vi "HFRR ADV v03.vi"() -> ()   [LabVIEW 2025] (continued)
            n807 = call "CAMERA LIVE FEED FGV.vi"("Enum - Menu"=CAMERA_LIVE_FEED_ENUM."CAMERA MINIMIZE") -> ()  [unwired: 9 in, 2 out]
          }
        }
        n808 = local write "CAMERA ROI MAX TEMP"(TRUE ("CAMERA ROI MAX TEMP")) -> ()
        n809 = case shown="True" w1172 {
          selector: w1172 -> [_ w1178]
          frame False {
          }
          frame True {
            n810 = Not(x=w1178) -> (.not. x?=w1177:bool)
            n811 = local write "CAMERA ROI MIN TEMP"(w1177) -> ()
            n812 = call "IMAGE ANALYSIS.vi"("Enum"=POST_ANALYSIS_ENUM."MINIMIZE UI") -> ()  [unwired: 9 in, 2 out]
          }
        }
      }
      frame "Mooha" {
        n813 = local read "LIVE FEED MIN TEMP"() -> (w1184:bool)
        n814 = local write "LIVE FEED MAX TEMP"(TRUE ("LIVE FEED MAX TEMP")) -> ()
        n815 = local read "CAMERA ROI MIN TEMP"() -> (w1182:bool)
        n816 = case shown="True" w1184 {
          selector: w1184 -> [_ w1191]
          frame False {
          }
          frame True {
            n817 = Not(x=w1191) -> (.not. x?=w1190:bool)
            n818 = local write "LIVE FEED MIN TEMP"(w1190) -> ()
            n819 = call "CAMERA LIVE FEED FGV.vi"("Enum - Menu"=CAMERA_LIVE_FEED_ENUM."CAMERA MINIMIZE") -> ()  [unwired: 9 in, 2 out]
          }
        }
        n820 = local write "CAMERA ROI MAX TEMP"(TRUE ("CAMERA ROI MAX TEMP")) -> ()
        n821 = case shown="True" w1182 {
          selector: w1182 -> [_ w1188]
          frame False {
          }
          frame True {
            n822 = Not(x=w1188) -> (.not. x?=w1187:bool)
            n823 = local write "CAMERA ROI MIN TEMP"(w1187) -> ()
            n824 = call "IMAGE ANALYSIS.vi"("Enum"=POST_ANALYSIS_ENUM."MINIMIZE UI") -> ()  [unwired: 9 in, 2 out]
          }
        }
      }
    }
    n825 = local read "Auto Start Test"() -> (w933:bool)
    n826 = case shown="True" "sign in temp" {
      frame False {
      }
      frame True {
        w970 = 1 ("y")
        n827 = local read "USERNAME"() -> (w976:string)
        n828 = local read "USER ID"() -> (w973:string)
        n829 = call <vilib>:"Trim Whitespace.vi"("string"=w976) -> ("trimmed string"=w975:string)  [unwired: 1 in]
        n830 = call <vilib>:"Trim Whitespace.vi"("string"=w973) -> ("trimmed string"=w974:string)  [unwired: 1 in]
        n831 = String Length(string=w975) -> (length=w972:i32)
        n832 = String Length(string=w974) -> (length=w971:i32)
        n833 = Greater?(x=w972, y=w970) -> (0:w969:bool)
        n834 = Greater?(x=w971, y=w970) -> (0:w968:bool)
        n835 = And(x=w969, y=w968) -> (x .and. y?=w967:bool)
        n836 = case shown="True" w967 {
          frame False {
            n837 = property on="Sign In" class="Bool (strict)"("DisabledEnum"=T13."Disabled" ("Disabled")) -> ()  [unwired: 2 in, 2 out]
          }
          frame True {
            n838 = property on="Sign In" class="Bool (strict)"("DisabledEnum"=T13."Enabled" ("Disabled")) -> ()  [unwired: 2 in, 2 out]
          }
        }
      }
    }
    n839 = local read "Air Temperature"() -> (w950:bool)
    n840 = local read "Coefficient Of Friction"() -> (w951:bool)
    n841 = case shown="False" w933 {
      frame False {
        n842 = local read "Auto stop temp"() -> (w964:bool)
        n843 = case shown="True" w964 {
          frame False {
          }
          frame True {
            n844 = local write "Auto Start Temp"(FALSE ("Auto Start Temp")) -> ()
          }
        }
      }
      frame True {
        "Auto stop temp" <- TRUE ("Auto stop temp")
      }
    }
    n845 = local read "Humidity"() -> (w949:bool)
    n846 = case shown="\"HOME\"" w961 {
      frame "HOME" {
        n847 = local write "main tab sub"(enum32{"Page 1", "Page 2"}."Page 1" ("main tab sub")) -> ()
      }
      frame Default {
        n848 = local write "main tab sub"(enum32{"Page 1", "Page 2"}."Page 2" ("main tab sub")) -> ()
      }
    }
    n849 = case shown="True" w960 {
      selector: w960 -> [_ w1296]
      frame False {
      }
      frame True {
        n850 = Not(x=w1296) -> (.not. x?=w1295:bool)
        n851 = local write "Sign In"(w1295) -> ()
        n852 = local write "Main Dashboard Buttons"(T1."Test Setup" ("Main Dashboard Buttons")) -> ()
      }
    }
    n853 = case shown="\"Numeric Display\", Default" "Num/Graph" {
      frame "Numeric Display", Default {
        n854 = property on="Single/Multiple" class="RadioBtnsControl (strict)"("Visible"=FALSE) -> ()  [unwired: 2 in, 2 out]
        n855 = property on="Single - Graph" class="Ring (strict)"("Visible"=FALSE) -> ()  [unwired: 2 in, 2 out]
        n856 = local write "Main Tab Display"(T4."Dashboard 1" ("Main Tab Display")) -> ()
      }
      frame "Graph Display" {
        n857 = property on="Single/Multiple" class="RadioBtnsControl (strict)"("Visible"=TRUE) -> ()  [unwired: 2 in, 2 out]
        n858 = case shown="\"Multiple\"" "Single/Multiple" {
          frame "Single ", Default {
            n859 = property on="Single - Graph" class="Ring (strict)"("Visible"=TRUE) -> ()  [unwired: 2 in, 2 out]
            n860 = local write "Main Tab Display"(T4."Dashboard 3" ("Main Tab Display")) -> ()
          }
          frame "Multiple" {
            n861 = property on="Single - Graph" class="Ring (strict)"("Visible"=FALSE) -> ()  [unwired: 2 in, 2 out]
            n862 = local write "Main Tab Display"(T4."Dashboard 2" ("Main Tab Display")) -> ()
          }
        }
      }
    }
    n863 = local read "Stroke"() -> (w948:bool)
    n864 = local read "USERNAME"() -> (w954:string)
    n865 = local read "USER ID"() -> (w953:string)
    n866 = case shown="True" w951 {
      selector: w951 -> [_ w1231]
      frame False {
      }
      frame True {
        n867 = Not(x=w1231) -> (.not. x?=w1230:bool)
        n868 = local write "Coefficient Of Friction"(w1230) -> ()
        n869 = local write "Tab Control 2"(T6."Coefficient Of Friction" ("Tab Control 2")) -> ()
      }
    }
    n870 = case shown="True" w950 {
      selector: w950 -> [_ w1228]
      frame False {
      }
      frame True {
        n871 = Not(x=w1228) -> (.not. x?=w1226:bool)
        n872 = local write "Air Temperature"(w1226) -> ()
        n873 = local write "Tab Control 2"(T6."Air Temperature" ("Tab Control 2")) -> ()
      }
    }
    n874 = local write "Operator ID"(w953) -> ()
    n875 = case shown="True" w948 {
      selector: w948 -> [_ w1222]
      frame False {
      }
      frame True {
        n876 = Not(x=w1222) -> (.not. x?=w1220:bool)
        n877 = local write "Stroke"(w1220) -> ()
        n878 = local write "Tab Control 2"(T6."Stroke" ("Tab Control 2")) -> ()
      }
    }
    n879 = local write "tested by"(w954) -> ()
    n880 = case shown="True" w949 {
      selector: w949 -> [_ w1225]
      frame False {
      }
      frame True {
        n881 = Not(x=w1225) -> (.not. x?=w1223:bool)
        n882 = local write "Humidity"(w1223) -> ()
        n883 = local write "Tab Control 2"(T6."Humidity" ("Tab Control 2")) -> ()
      }
    }
    n884 = case shown="\"Advance\"" "Main Dashboard Buttons" {
      tunnel: [T2."HOME" ("Main Tab") T2."Test Setup" ("Main Tab") T2."Acquire" ("Main Tab") T2."Adv Scar" ("Main Tab") T2."Adv Scar Report" ("Main Tab") T2."Compare Files" ("Main Tab") T2."About" ("Main Tab") T2."Advance" ("Main Tab")] -> w958
      frame "Home", Default {
      }
      frame "Test Setup" {
      }
      frame "Dashboard" {
      }
      frame "Imaging" {
      }
      frame "Report" {
      }
      frame "Analysis" {
      }
      frame "About" {
      }
      frame "Advance" {
      }
    }
    n885 = Wait (ms)(milliseconds to wait=u32 100) -> ()  [unwired: 1 out]
    n886 = local read "Main Tab Display"() -> (w952:T4)
    n887 = local write "Main Tab"(w958) -> ()
    n888 = case shown="\"Dashboard 3\"" w952 {
      frame "Dashboard 1", Default {
        n889 = property on="Reset Graph" class="Bool (strict)"("Visible"=FALSE) -> ()  [unwired: 2 in, 2 out]
      }
      frame "Dashboard 2" {
        n890 = property on="Reset Graph" class="Bool (strict)"("Visible"=TRUE) -> ()  [unwired: 2 in, 2 out]
      }
      frame "Dashboard 3" {
        n891 = property on="Reset Graph" class="Bool (strict)"("Visible"=TRUE) -> ()  [unwired: 2 in, 2 out]
      }
    }
    n892 = local read "SCAR MEASURMENT"() -> (w940:enum32{"Auto Scar", "Manual Scar"})
    n893 = local read "Humidity"() -> (w955:bool)
    n894 = local read "Cap Live Image"() -> (w937:bool)
    n895 = local read "Sample Temperature"() -> (w947:bool)
    n896 = local read "Air Temp vs Humidity"() -> (w945:bool)
    n897 = local read "Frequency"() -> (w946:bool)
    n898 = case shown="False" w955 {
      frame False {
        n899 = local write "Humidity On Command"(TRUE ("Humidity On Command")) -> ()
        n900 = case shown="True" "Humidity Off Command" {
          selector: "Humidity Off Command" -> [_ w1238]
          frame False {
          }
          frame True {
            n901 = stacked-sequence {
              frame #0 {
                n902 = local read "WriteHumidity"() -> (w1240:string[])
                n903 = Insert Into Array(array=w1240, new element="R;1" ("new element/subarray")) -> (w1241:string[])  [unwired: 1 in]
                n904 = local write "WriteHumidity"(w1241) -> ()
              }
              frame #1 {
                n905 = Wait (ms)(milliseconds to wait=u32 2000) -> ()  [unwired: 1 out]
              }
              frame #2 {
                n906 = local read "EVENT LOG"() -> (w1247:string)
                n907 = local read "WriteHumidity"() -> (w1244:string[])
                n908 = call "Event Log.vi"("Content"="Humidity Control Off" ("string"), "EVENT LOG"=w1247) -> ("EVENT LOG"=w1248:string)  [unwired: 8 in, 1 out]
                n909 = local write "EVENT LOG"(w1248) -> ()
                n910 = Insert Into Array(array=w1244, new element="R;1" ("new element/subarray")) -> (w1245:string[])  [unwired: 1 in]
                n911 = local write "WriteHumidity"(w1245) -> ()
              }
            }
            n912 = Not(x=w1238) -> (.not. x?=w1237:bool)
            n913 = local write "Humidity Off Command"(w1237) -> ()
          }
        }
      }
      frame True {
        n914 = local write "Humidity Off Command"(TRUE ("Humidity Off Command")) -> ()
        n915 = case shown="False" "Humidity On Command" {
          selector: "Humidity On Command" -> [_ w1252]
          frame False {
          }
          frame True {
            n916 = stacked-sequence {
              frame #0 {
                n917 = local read "Set Rh"() -> (w1258:dbl)
                n918 = Number To Fractional String(number=w1258, precision (6)=i16 2) -> (F-format string=w1259:string)  [unwired: 2 in]
                n919 = local read "WriteHumidity"() -> (w1256:string[])
                n920 = Concatenate Strings("M;" ("new element/subarray"), w1259) -> (w1257:string)
                n921 = Insert Into Array(array=w1256, new element=w1257) -> (w1255:string[])  [unwired: 1 in]
                n922 = local write "WriteHumidity"(w1255) -> ()
              }
              frame #1 {
                n923 = Wait (ms)(milliseconds to wait=u32 1500) -> ()  [unwired: 1 out]
              }
              frame #2 {
                (unwired) "% RH" ("string")
                (unwired) i16 2 ("precision (6)")
                (unwired) "M;" ("new element/subarray")
                n924 = local read "Set Rh"() -> (w1266:dbl)
                n925 = Number To Fractional String(number=w1266, precision (6)=i16 2) -> (F-format string=w1263:string)  [unwired: 2 in]
                n926 = local read "WriteHumidity"() -> (w1268:string[])
                n927 = Concatenate Strings("M;" ("new element/subarray"), w1263) -> (w1267:string)
                n928 = Concatenate Strings("Humidity Set to : " ("string"), w1263, "% RH" ("string")) -> (w1261:string)
                n929 = Insert Into Array(array=w1268, new element=w1267) -> (w1269:string[])  [unwired: 1 in]
                n930 = disable-structure shown="Enabled" {
                  frame Enabled {
                    n931 = local read "EVENT LOG"() -> (w1272:string)
                    n932 = call "Event Log.vi"("Content"="Humidity Control On", "EVENT LOG"=w1272) -> ("EVENT LOG"=w1273:string)  [unwired: 8 in, 1 out]
                    n933 = local write "EVENT LOG"(w1273) -> ()
                  }
                  frame Disabled {
                  }
                }
                n934 = disable-structure shown="Enabled" {
                  disable-tunnel: w1261 -> [_ _]
                  frame Enabled {
                    n935 = local read "EVENT LOG"() -> (w1275:string)
                    n936 = call "Event Log.vi"("Content"="Humidity Control On", "EVENT LOG"=w1275) -> ("EVENT LOG"=w1276:string)  [unwired: 8 in, 1 out]
                    n937 = local write "EVENT LOG"(w1276) -> ()
                  }
                  frame Disabled {
                  }
                }
                n938 = local write "WriteHumidity"(w1269) -> ()
              }
            }
            n939 = Not(x=w1252) -> (.not. x?=w1251:bool)
            n940 = local write "Humidity On Command"(w1251) -> ()
          }
        }
      }
    }
    n941 = Equal?(x=w940, y=enum32{"Auto Scar", "Manual Scar"}."Auto Scar" ("SCAR MEASURMENT")) -> (x = y?=w936:bool)
    n942 = local read "TEST STANDARD"() -> (w943:T3)
    n943 = And(x=w937, y=w936) -> (x .and. y?=w938:bool)
    n944 = case shown="True" w938 {
      selector: w938 -> [_ w1037]
      tunnel: errorcluster {"status"=FALSE, "code"=0, "source"=""} ("error in (no error) 3") -> [_ w1038]
      frame False {
      }
      frame True {
        n945 = stacked-sequence {
          tunnel: w1038 -> [_ _ _ _ _ _ _ w1086]
          tunnel: w1037 -> [_ _ _ _ _ w1067 _ _]
          frame #0 {
            n946 = call "CAMERA LIVE FEED FGV.vi"("Enum - Menu"=CAMERA_LIVE_FEED_ENUM."CAMERA MINIMIZE") -> ()  [unwired: 9 in, 2 out]
          }
          frame #1 {
            n947 = property on="Auto Scar Check  2" class="Clust (strict)"("Visible"=TRUE) -> ()  [unwired: 2 in, 2 out]
          }
          frame #2 {
            n948 = String To Path(string="C:\\LAB-IQ\\Image Calibrate v01.dcf") -> (path=w1043:path)
            n949 = Open/Create/Replace File ("Open File")(file path (use dialog)=w1043) -> (refnum out=w1044:refnum<file>)  [unwired: 5 in, 2 out]
            n950 = for {
              N: 4 -> [_]
              tunnel: w1044 -> [w1050]
              i -> [w1046]
              n951 = Read from Text File ("Read File")(file (use dialog)=w1050) -> (text=w1051:string)  [unwired: 3 in, 3 out]
              n952 = String Subset(string=w1051, offset (0)=6, length (rest)=10 ("length (rest)")) -> (substring=w1047:string)
              n953 = Fract/Exp String To Number(string=w1047) -> (number=w1045:dbl)  [unwired: 3 in, 1 out]
              n954 = case shown="0" w1046 {
                tunnel: w1045 -> [w1052 w1053 _ w1054 _]
                frame 0 {
                  "5x Gain" <- w1052
                }
                frame 1 {
                  "10x Gain" <- w1053
                }
                frame 2 {
                }
                frame 3 {
                  "100x gain" <- w1054
                }
                frame 4, Default {
                }
              }
            }
          }
          frame #3 {
            n955 = local read "FILE 3"() -> (w1060:string)
            n956 = call <vilib>:"Trim Whitespace.vi"("string"="C:\\LAB-IQ\\images\\") -> ("trimmed string"=w1062:string)  [unwired: 1 in]
            n957 = String To Path(string=w1062) -> (path=w1061:path)
            n958 = Concatenate Strings(w1060, ".png" ("string")) -> (w1059:string)
            n959 = Build Path(base path=w1061, name or relative path=w1059) -> (appended path=w1057:path)
            "Image path" <- w1057
            n960 = Path To String(path=w1057) -> (string=w1056:string)
            n961 = call "CAMERA LIVE FEED FGV.vi"("Enum - Menu"=CAMERA_LIVE_FEED_ENUM."CAMERA SAVE", "Image Path"=w1056) -> ()  [unwired: 8 in, 2 out]
          }
          frame #4 {
            n962 = One Button Dialog(message="Image saved successfully") -> ()  [unwired: 1 in, 1 out]
          }
          frame #5 {
            n963 = local read "TEST STANDARD"() -> (w1066:T3)
            n964 = local read "Magnification len live scar"() -> (w1078:string)
            n965 = Not(x=w1067) -> (.not. x?=w1068:bool)
            n966 = local write "Cap Live Image"(w1068) -> ()
            n967 = case shown="\"ISO 12156\"" w1066 {
              tunnel: ["ASTM D6079" "ISO 12156"] -> w1065
              frame "ASTM D6079", Default {
              }
              frame "ISO 12156" {
              }
            }
            n968 = case shown="\"5x\", Default" w1078 {
              tunnel: [w1081 w1082] -> w1077
              frame "5x", Default {
                n969 = local read "5x Gain"() -> (w1081:dbl)
              }
              frame "10x" {
                # "5x"
                n970 = local read "10x Gain"() -> (w1082:dbl)
              }
            }
            n971 = local read "Image path"() -> (w1076:path)
            n972 = local read "FILE 3"() -> (w1069:string)
            n973 = call "EDGE DETCTION.vi"("GAIN VALUE"=w1077, "Image Path"=w1076) -> ("error out"=w1075:errorcluster, "return value"=w1074:cluster{string, string, dbl, dbl, dbl})  [unwired: 8 in]
            n974 = Bundle By Name(cluster=T18 {"File Name"="", "Test Method"="", "Operator"="", "Fuel Description"="", "Date and time"=""} ("Main Ref"), "File Name"=w1069, "Test Method"=w1065) -> (w1070:T18)
            n975 = call "duf file read.vi"("error in (no error)"=w1075, "Main Ref"=w1070) -> ("error out"=w1073:errorcluster, "Main Ref 2"=w1071:T18)  [unwired: 8 in]
            n976 = call "EDGE DETECTION REPORT.vi"("error in (no error)"=w1073, "return value 2"=w1074, "Main Ref"=w1071) -> ()  [unwired: 8 in, 1 out]
          }
          frame #6 {
            n977 = property on="Auto Scar Check  2" class="Clust (strict)"("Visible"=FALSE) -> ()  [unwired: 2 in, 2 out]
          }
          frame #7 {
            n978 = call "CAMERA LIVE FEED FGV.vi"("Enum - Menu"=CAMERA_LIVE_FEED_ENUM."CAMERA MINIMIZE", "error in (no error)"=w1086) -> ()  [unwired: 8 in, 2 out]
            n979 = local write "Main Dashboard Buttons"(T1."Home" ("Main Dashboard Buttons")) -> ()
            n980 = local write "Main Tab"(T2."HOME" ("Main Tab")) -> ()
          }
        }
      }
    }
    n981 = local read "Heater Button"() -> (w944:bool)
    n982 = case shown="True" w946 {
      selector: w946 -> [_ w1216]
      frame False {
      }
      frame True {
        n983 = Not(x=w1216) -> (.not. x?=w1214:bool)
        n984 = local write "Frequency"(w1214) -> ()
        n985 = local write "Tab Control 2"(T6."Frequency" ("Tab Control 2")) -> ()
      }
    }
    n986 = case shown="True" w945 {
      selector: w945 -> [_ w1213]
      frame False {
      }
      frame True {
        n987 = Not(x=w1213) -> (.not. x?=w1211:bool)
        n988 = local write "Air Temp vs Humidity"(w1211) -> ()
        n989 = local write "Tab Control 2"(T6."Air Temp vs Rh" ("Tab Control 2")) -> ()
      }
    }
    n990 = case shown="True" w947 {
      selector: w947 -> [_ w1219]
      frame False {
      }
      frame True {
        n991 = Not(x=w1219) -> (.not. x?=w1217:bool)
        n992 = local write "Sample Temperature"(w1217) -> ()
        n993 = local write "Tab Control 2"(T6."Sample Temperature" ("Tab Control 2")) -> ()
      }
    }
    n994 = case shown="\"Custom\"" w943 {
      frame "ASTM D6079", Default {
        w1192 = "ASTM D6079 TEST CONDITIONS" ("Standard 2")
        n995 = local write "Standard 2"(w1192) -> ()
        n996 = local write "Standard"(w1192) -> ()
      }
      frame "ISO 12156" {
        w1193 = "ISO 12156 TEST CONDITIONS" ("Standard 2")
        n997 = local write "Standard 2"(w1193) -> ()
        n998 = local write "Standard"(w1193) -> ()
      }
      frame "CEC F-096-A-06" {
        w1194 = "CEC F-096-A-06 TEST CONDITIONS" ("Standard 2")
        n999 = local write "Standard 2"(w1194) -> ()
        n1000 = local write "Standard"(w1194) -> ()
      }
      frame "Custom" {
        w1195 = "CUSTOM TEST CONDITIONS" ("Standard 2")
        n1001 = local write "Standard 2"(w1195) -> ()
        n1002 = local write "Standard"(w1195) -> ()
      }
    }
    n1003 = case shown="True" w944 {
      frame False {
        n1004 = local write "Temperature On Command"(TRUE ("Temperature On Command")) -> ()
        n1005 = case shown="True" "Temperature Off Command" {
          selector: "Temperature Off Command" -> [_ w1199]
          frame False {
          }
          frame True {
            n1006 = Not(x=w1199) -> (.not. x?=w1198:bool)
            n1007 = local read "EVENT LOG"() -> (w1202:string)
            n1008 = local write "Temperature Off Command"(w1198) -> ()
            n1009 = call "Event Log.vi"("Content"="Heater Off", "EVENT LOG"=w1202) -> ("EVENT LOG"=w1201:string)  [unwired: 8 in, 1 out]
            n1010 = local write "EVENT LOG"(w1201) -> ()
          }
        }
      }
      frame True {
        n1011 = local write "Temperature Off Command"(TRUE ("Temperature Off Command")) -> ()
        n1012 = case shown="True" "Temperature On Command" {
          selector: "Temperature On Command" -> [_ w1206]
          frame False {
          }
          frame True {
            n1013 = Not(x=w1206) -> (.not. x?=w1205:bool)
            n1014 = local write "Temperature On Command"(w1205) -> ()
            n1015 = disable-structure shown="Enabled" {
              disable-tunnel: "Heater On" -> [w1208 _]
              frame Enabled {
                n1016 = local read "EVENT LOG"() -> (w1209:string)
                n1017 = call "Event Log.vi"("Content"=w1208, "EVENT LOG"=w1209) -> ("EVENT LOG"=w1210:string)  [unwired: 8 in, 1 out]
                n1018 = local write "EVENT LOG"(w1210) -> ()
              }
              frame Disabled {
              }
            }
          }
        }
      }
    }
    n1019 = local read "Main Tab"() -> (w935:T2)
    n1020 = case shown="\"About\"" w935 {
      frame "HOME", Default {
        w981 = T13."Enabled" ("Disabled")
        n1021 = local read "Service Password enable"() -> (w980:bool)
        n1022 = property on="Imaging" class="Bool (strict)"("DisabledEnum"=w981) -> ()  [unwired: 2 in, 2 out]
        n1023 = property on="Dashboard" class="Bool (strict)"("DisabledEnum"=w981) -> ()  [unwired: 2 in, 2 out]
        n1024 = property on="Test Setup" class="Bool (strict)"("DisabledEnum"=w981) -> ()  [unwired: 2 in, 2 out]
        n1025 = property on="Analysis" class="Bool (strict)"("DisabledEnum"=w981) -> ()  [unwired: 2 in, 2 out]
        n1026 = property on="Home" class="Bool (strict)"("DisabledEnum"=w981) -> ()  [unwired: 2 in, 2 out]
        n1027 = property on="Report" class="Bool (strict)"("DisabledEnum"=w981) -> ()  [unwired: 2 in, 2 out]
        n1028 = property on="Main Dashboard Buttons" class="RadioBtnsControl (strict)"("DisabledEnum"=w981) -> ()  [unwired: 2 in, 2 out]
        n1029 = case shown="True" w980 {
          tunnel: [T13."Disabled" ("Disabled") T13."Enabled" ("Disabled")] -> w979
          frame False {
          }
          frame True {
          }
        }
        n1030 = property on="About" class="Bool (strict)"("DisabledEnum"=w979) -> ()  [unwired: 2 in, 2 out]
      }
      frame "Test Setup" {
        w986 = T13."Enabled" ("Disabled")
        n1031 = local read "Service Password enable"() -> (w985:bool)
        n1032 = property on="Dashboard" class="Bool (strict)"("DisabledEnum"=T13."Disabled" ("Disabled")) -> ()  [unwired: 2 in, 2 out]
        n1033 = property on="Imaging" class="Bool (strict)"("DisabledEnum"=w986) -> ()  [unwired: 2 in, 2 out]
        n1034 = property on="Analysis" class="Bool (strict)"("DisabledEnum"=w986) -> ()  [unwired: 2 in, 2 out]
        n1035 = property on="Home" class="Bool (strict)"("DisabledEnum"=w986) -> ()  [unwired: 2 in, 2 out]
        n1036 = property on="Report" class="Bool (strict)"("DisabledEnum"=w986) -> ()  [unwired: 2 in, 2 out]
        n1037 = property on="Test Setup" class="Bool (strict)"("DisabledEnum"=w986) -> ()  [unwired: 2 in, 2 out]
        n1038 = case shown="True" w985 {
          tunnel: [T13."Disabled" ("Disabled") T13."Enabled" ("Disabled")] -> w984
          frame False {
          }
          frame True {
          }
        }
        n1039 = property on="About" class="Bool (strict)"("DisabledEnum"=w984) -> ()  [unwired: 2 in, 2 out]
      }
      frame "Adv Scar" {
        w993 = T13."Enabled" ("Disabled")
        n1040 = property on="Dashboard" class="Bool (strict)"("DisabledEnum"=T13."Disabled" ("Disabled")) -> ()  [unwired: 2 in, 2 out]
        n1041 = property on="Imaging" class="Bool (strict)"("DisabledEnum"=w993) -> ()  [unwired: 2 in, 2 out]
        n1042 = property on="Analysis" class="Bool (strict)"("DisabledEnum"=w993) -> ()  [unwired: 2 in, 2 out]
        n1043 = property on="Home" class="Bool (strict)"("DisabledEnum"=w993) -> ()  [unwired: 2 in, 2 out]
        n1044 = property on="Report" class="Bool (strict)"("DisabledEnum"=w993) -> ()  [unwired: 2 in, 2 out]
        n1045 = property on="Test Setup" class="Bool (strict)"("DisabledEnum"=w993) -> ()  [unwired: 2 in, 2 out]
        n1046 = local read "Service Password enable"() -> (w991:bool)
        n1047 = case shown="True" w991 {
          tunnel: [T13."Disabled" ("Disabled") T13."Enabled" ("Disabled")] -> w990
          frame False {
          }
          frame True {
          }
        }
        n1048 = property on="About" class="Bool (strict)"("DisabledEnum"=w990) -> ()  [unwired: 2 in, 2 out]
      }
      frame "Adv Scar Report" {
        w998 = T13."Enabled" ("Disabled")
        n1049 = property on="Dashboard" class="Bool (strict)"("DisabledEnum"=T13."Disabled" ("Disabled")) -> ()  [unwired: 2 in, 2 out]
        n1050 = property on="Imaging" class="Bool (strict)"("DisabledEnum"=w998) -> ()  [unwired: 2 in, 2 out]
        n1051 = property on="Analysis" class="Bool (strict)"("DisabledEnum"=w998) -> ()  [unwired: 2 in, 2 out]
        n1052 = property on="Home" class="Bool (strict)"("DisabledEnum"=w998) -> ()  [unwired: 2 in, 2 out]
        n1053 = property on="Report" class="Bool (strict)"("DisabledEnum"=w998) -> ()  [unwired: 2 in, 2 out]
        n1054 = property on="Test Setup" class="Bool (strict)"("DisabledEnum"=w998) -> ()  [unwired: 2 in, 2 out]
        n1055 = local read "Service Password enable"() -> (w997:bool)
        n1056 = case shown="True" w997 {
          tunnel: [T13."Disabled" ("Disabled") T13."Enabled" ("Disabled")] -> w996
          frame False {
          }
          frame True {
          }
        }
        n1057 = property on="About" class="Bool (strict)"("DisabledEnum"=w996) -> ()  [unwired: 2 in, 2 out]
      }
      frame "Compare Files" {
        w1004 = T13."Enabled" ("Disabled")
        n1058 = local read "Service Password enable"() -> (w1003:bool)
        n1059 = property on="Dashboard" class="Bool (strict)"("DisabledEnum"=T13."Disabled" ("Disabled")) -> ()  [unwired: 2 in, 2 out]
        n1060 = property on="Imaging" class="Bool (strict)"("DisabledEnum"=w1004) -> ()  [unwired: 2 in, 2 out]
        n1061 = property on="Analysis" class="Bool (strict)"("DisabledEnum"=w1004) -> ()  [unwired: 2 in, 2 out]
        n1062 = property on="Home" class="Bool (strict)"("DisabledEnum"=w1004) -> ()  [unwired: 2 in, 2 out]
        n1063 = property on="Report" class="Bool (strict)"("DisabledEnum"=w1004) -> ()  [unwired: 2 in, 2 out]
        n1064 = property on="Test Setup" class="Bool (strict)"("DisabledEnum"=w1004) -> ()  [unwired: 2 in, 2 out]
        n1065 = case shown="True" w1003 {
          tunnel: [T13."Disabled" ("Disabled") T13."Enabled" ("Disabled")] -> w1002
          frame False {
          }
          frame True {
          }
        }
        n1066 = property on="About" class="Bool (strict)"("DisabledEnum"=w1002) -> ()  [unwired: 2 in, 2 out]
      }
      frame "Acquire" {
        n1067 = local read "Service Password enable"() -> (w1008:bool)
        n1068 = property on="Test Setup" class="Bool (strict)"("DisabledEnum"=T13."Disabled" ("Disabled")) -> ()  [unwired: 2 in, 2 out]
        n1069 = local read "Auto Start Test"() -> (w1010:bool)
        n1070 = local read "RUN"() -> (w1012:bool)
        n1071 = case shown="True" w1008 {
          tunnel: [T13."Disabled" ("Disabled") T13."Enabled" ("Disabled")] -> w1009
          frame False {
          }
          frame True {
          }
        }
        n1072 = Or(x=w1012, y=w1010) -> (x .or. y?=w1011:bool)
        n1073 = case shown="True" w1011 {
          tunnel: [T13."Enabled" ("Disabled") T13."Disabled" ("Disabled")] -> w1014
          frame False {
          }
          frame True {
          }
        }
        n1074 = property on="About" class="Bool (strict)"("DisabledEnum"=w1009) -> ()  [unwired: 2 in, 2 out]
        n1075 = property on="Imaging" class="Bool (strict)"("DisabledEnum"=w1014) -> ()  [unwired: 2 in, 2 out]
        n1076 = property on="Dashboard" class="Bool (strict)"("DisabledEnum"=w1014) -> ()  [unwired: 2 in, 2 out]
        n1077 = property on="Analysis" class="Bool (strict)"("DisabledEnum"=w1014) -> ()  [unwired: 2 in, 2 out]
        n1078 = property on="Home" class="Bool (strict)"("DisabledEnum"=w1014) -> ()  [unwired: 2 in, 2 out]
        n1079 = property on="Report" class="Bool (strict)"("DisabledEnum"=w1014) -> ()  [unwired: 2 in, 2 out]
      }
      frame "About" {
        n1080 = local read "FILE"() -> (w1027:string)
        n1081 = local read "TEST FILE NAM,E SAVED"() -> (w1020:bool)
        n1082 = call <vilib>:"Trim Whitespace.vi"("string"=w1027) -> ("trimmed string"=w1026:string)  [unwired: 1 in]
        n1083 = local read "Auto Start Test"() -> (w1030:bool)
        n1084 = String Length(string=w1026) -> (length=w1025:i32)
        n1085 = Greater?(x=w1025, y=1) -> (0:w1022:bool)
        n1086 = And(x=w1022, y=w1020) -> (x .and. y?=w1021:bool)
        n1087 = local read "RUN"() -> (w1032:bool)
        n1088 = case shown="True" w1021 {
          tunnel: [T13."Disabled" ("Disabled") T13."Enabled" ("Disabled")] -> w1023
          frame False {
          }
          frame True {
          }
        }
        n1089 = Or(x=w1032, y=w1030) -> (x .or. y?=w1031:bool)
        n1090 = property on="About" class="Bool (strict)"("DisabledEnum"=T13."Enabled" ("Disabled")) -> ()  [unwired: 2 in, 2 out]
        n1091 = case shown="False" w1031 {
          tunnel: [T13."Enabled" ("Disabled") T13."Disabled" ("Disabled")] -> w1029
          frame False {
          }
          frame True {
          }
        }
        n1092 = property on="Dashboard" class="Bool (strict)"("DisabledEnum"=w1023) -> ()  [unwired: 2 in, 2 out]
        n1093 = property on="Test Setup" class="Bool (strict)"("DisabledEnum"=T13."Disabled" ("Disabled")) -> ()  [unwired: 2 in, 2 out]
        n1094 = property on="Imaging" class="Bool (strict)"("DisabledEnum"=w1029) -> ()  [unwired: 2 in, 2 out]
        n1095 = property on="Analysis" class="Bool (strict)"("DisabledEnum"=w1029) -> ()  [unwired: 2 in, 2 out]
        n1096 = property on="Home" class="Bool (strict)"("DisabledEnum"=w1029) -> ()  [unwired: 2 in, 2 out]
        n1097 = property on="Report" class="Bool (strict)"("DisabledEnum"=w1029) -> ()  [unwired: 2 in, 2 out]
      }
    }
    n1098 = local read "Quit"() -> (w963:bool)
    "Single" <- "Single - Graph"
  }
  n1099 = disable-structure shown="Disabled" {
    disable-tunnel: [w1300 _] -> w39
    disable-tunnel: _ -> [w1299 _]
    frame Disabled {
      n1100 = while {
        tunnel: w1299 -> [_]
        tunnel: [w1301] -> w1300
        tunnel: [w1302] -> _
        i -> [w1302]
        stop <- w1301 stop-if-true
        w1318 = u16 10 items=["1.0"=10, "1.5"=15, "2.0"=20] ("stop bits (10: 1 bit)")
        n1101 = Wait (ms)(milliseconds to wait=u32 10) -> ()  [unwired: 1 out]
        n1102 = call-poly "VISA Configure Serial Port"("VISA resource name"=refnum<visa-resource-name> "ASRL1::INSTR" ("COM PORT"), "timeout (10sec)"=u32 10, "baud rate (9600)"=u32 57600, "data bits (8)"=u16 8, "stop bits (10: 1 bit)"=w1318) -> ("VISA resource name out"=w1304:refnum<visa-resource-name>, "error out"=w1313:errorcluster)  [unwired: 9 in]
        n1103 = VISA Read(VISA resource name=w1304, byte count=u32 2 ("byte count (0)")) -> (read buffer=w1312:string)  [unwired: 1 in, 3 out]
        n1104 = String Subset(string=w1312, offset (0)=0, length (rest)=2 ("length (rest)")) -> (substring=w1311:string)
        n1105 = Match Pattern(string=w1311, regular expression="<>") -> (offset past match=w1308:i32)  [unwired: 1 in, 3 out]
        n1106 = Greater Or Equal?(x=w1308, y=0) -> (x >= y?=w1303:bool)
        n1107 = case shown="True" w1303 {
          tunnel: w1304 -> [_ w1322]
          tunnel: w1313 -> [_ w1321]
          frame False {
          }
          frame True {
            n1108 = VISA Read(VISA resource name=w1322, byte count=u32 32 ("byte count (0)"), error in (no error)=w1321) -> (read buffer=w1320:string)  [unwired: 3 out]
            n1109 = String Subset(string=w1320, offset (0)=0, length (rest)=8 ("length (rest)")) -> (substring=w1324:string)
            n1110 = String Subset(string=w1320, offset (0)=8, length (rest)=8 ("length (rest)")) -> (substring=w1325:string)
            n1111 = Decimal String To Number(string=w1325) -> (number=w1332:i32)  [unwired: 2 in, 1 out]
            n1112 = Decimal String To Number(string=w1324) -> (number=w1328:i32)  [unwired: 2 in, 1 out]
            n1113 = Divide(x=w1332, y=10000) -> ()  [unwired: 1 out]
            n1114 = Divide(x=w1328, y=1000000) -> ()  [unwired: 1 out]
          }
        }
        n1115 = local read "Quit"() -> (w1301:bool)
      }
    }
    frame Enabled {
    }
  }
  n1116 = while {
    shift-right: [w1347] -> w52
    shift-left: _ -> [w1338]
    shift-right: [w1346] -> w51
    shift-left: errorcluster {"status"=TRUE, "code"=0, "source"="Init"} ("error IO") -> [w1340]
    tunnel: [w1335] -> w42
    tunnel: [w1345] -> _
    i -> [w1345]
    stop <- w1335 stop-if-true
    n1117 = local read "Port 1a"() -> (w1341:bool)
    n1118 = local read "Port 3"() -> (w1342:bool)
    n1119 = local read "Com Port 1"() -> (w1339:refnum<visa-resource-name>)
    n1120 = Or(x=w1342, y=w1341) -> (x .or. y?=w1344:bool)
    n1121 = Unbundle(w1340) -> ("status"=→"Port 3":bool)  [unwired: 2 out]
    n1122 = Not Equal?(x=w1339, y=w1338) -> (x != y?=w1336:bool)
    n1123 = case shown="True" w1344 {
      frame False {
        w1350 = FALSE ("Visible")
        n1124 = property on="Port 1a" class="Bool (strict)"("Visible"=w1350) -> ()  [unwired: 2 in, 2 out]
        n1125 = property on="Port 3" class="Bool (strict)"("Visible"=w1350) -> ()  [unwired: 2 in, 2 out]
      }
      frame True {
        w1351 = TRUE ("Visible")
        n1126 = property on="Port 1a" class="Bool (strict)"("Visible"=w1351) -> ()  [unwired: 2 in, 2 out]
        n1127 = property on="Port 3" class="Bool (strict)"("Visible"=w1351) -> ()  [unwired: 2 in, 2 out]
      }
    }
    n1128 = Wait (ms)(milliseconds to wait=u32 10) -> ()  [unwired: 1 out]
    n1129 = case shown="True" w1336 {
      tunnel: [w1348 errorcluster {"status"=TRUE, "code"=0, "source"="Init"} ("error out")] -> w1337
      tunnel: w1340 -> [w1348 _]
      frame False {
      }
      frame True {
      }
    }
    n1130 = case shown="No Error" w1337 {
      selector: w1337 -> [w1358 w1385]
      tunnel: [w1361 w1389] -> w1347
      tunnel: [w1360 w1383] -> w1346
      tunnel: w1338 -> [w1359 w1387]
      frame No Error {
        n1131 = property class="Instr"(reference=w1359, error in=w1358) -> (reference out=w1356:refnum<visa-resource-name>, error out=w1357:errorcluster, "Serial Settings:Number of Bytes at Serial Port"=w1352:u32)
        n1132 = Greater?(x=w1352, y=u32 5) -> (0:w1354:bool)
        n1133 = Not(x=w1354) -> (.not. x?=→"Port 1a":bool)
        n1134 = while {
          tunnel: [w1378] -> w1360
          tunnel: [w1377] -> w1361
          tunnel: w1357 -> [w1376]
          tunnel: w1356 -> [w1375]
          stop <- TRUE stop-if-true
          n1135 = property class="Instr" props=["Serial Settings:Number of Bytes at Serial Port"](reference=w1375, error in=w1376) -> (reference out=w1380:refnum<visa-resource-name>, error out=w1379:errorcluster)  [unwired: 1 out]
          n1136 = VISA Read(VISA resource name=w1380, byte count=u32 1000, error in (no error)=w1379) -> (VISA resource name out=w1377:refnum<visa-resource-name>, read buffer=w1362:string, error out=w1378:errorcluster)  [unwired: 1 out]
          "UNI READ" <- w1362
          n1137 = Spreadsheet String To Array(delimiter (Tab)=";", format string="", spreadsheet string=w1362, array type (2D Dbl)=dbl[] []) -> (array=w1372:dbl[])
          n1138 = Index Array(array=w1372) -> (element #1=→"LVDT MIN":dbl, element #2=→"LVDT MAX":dbl, element #3=→"LVDT Peak":dbl, element #4=→"pizo raw":dbl, element #5=→"Friction":dbl, element #6=→"cof 2":dbl)  [unwired: 6 in]
        }
      }
      frame Error {
        w1395 = u16 0 items=["None", "XON/XOFF", "RTS/CTS", "XON/XOFF & RTS/CTS", "DTR/DSR", "XON/XOFF & DTR/DSR"] ("flow control (0:none)  2")
        w1393 = u16 10 items=["1.0"=10, "1.5"=15, "2.0"=20] ("stop bits 2")
        w1391 = u16 0 items=["None", "Odd", "Even", "Mark", "Space"] ("parity 2")
        w1392 = u32 10000  # timeout (10sec)
        n1139 = VISA Close(VISA resource name=w1387, error in (no error)=w1385) -> (error out=w1388:errorcluster)
        n1140 = local write "Port 1a"(FALSE ("Port 1a")) -> ()
        n1141 = local read "Com Port 1"() -> (w1382:refnum<visa-resource-name>)
        n1142 = call <vilib>:"Clear Errors.vi"("error in (no error)"=w1388) -> ("error out"=w1386:errorcluster)  [unwired: 5 in, 1 out]
        n1143 = call-poly "VISA Configure Serial Port"("VISA resource name"=w1382, "timeout (10sec)"=w1392, "baud rate (9600)"=u32 250000 ("baud rate  2"), "data bits (8)"=u16 8 ("data bits  2"), "parity (0:none)"=w1391, "error in (no error)"=w1386, "stop bits (10: 1 bit)"=w1393, "flow control (0:none)"=w1395) -> ("VISA resource name out"=w1396:refnum<visa-resource-name>, "error out"=w1397:errorcluster)  [unwired: 6 in]
        n1144 = flat-sequence {
          tunnel: w1396 -> [w1399]
          tunnel: w1397 -> [w1398]
          tunnel: [w1399] -> w1389
          tunnel: [w1398] -> w1383
          frame #0 {
            n1145 = Wait (ms)(milliseconds to wait=u32 50) -> ()  [unwired: 1 out]
          }
        }
        "Residual Uno" <- ""
        "Port 1 Error" <- w1383
      }
    }
    n1146 = local read "Quit"() -> (w1335:bool)
    "Error Uno" <- w1340
  }
  n1147 = while {
    stop <- w1406 stop-if-true
    # "V0OLTAGE TO STROKE (peice vise calibration)"
    n1148 = Wait (ms)(milliseconds to wait=u32 10) -> ()  [unwired: 1 out]
    n1149 = local read "LVDT Peak"() -> (w1403:dbl)
    n1150 = formula code="// Dynamic Parameterized Linear Interpolation Node\n// Inputs: vpp_val, voltages (Array), distances (Array)\n// Outputs: stroke\n\nint i = 0;\nint segments = 11; // 12 points make 11 interpolation segments\n\n// 1. Lower Boundary Clamp\nif (vpp_val <= voltages[0]) {\n    stroke = distances[0];\n}\n// 2. Upper Boundary Clamp\nelse if (vpp_val >= voltages[segments]) {\n    stroke = distances[segments];\n}\n// 3. Dynamic Segment Search Loop\nelse {\n    stroke = distances[0]; // Fallback baseline\n    for (i = 0; i < segments; i++) {\n        if (vpp_val >= voltages[i] && vpp_val <= voltages[i+1]) {\n            // Standard linear interpolation formula using array lookups\n            stroke = distances[i] + (vpp_val - voltages[i]) * (distances[i+1] - distances[i]) / (voltages[i+1] - voltages[i]);\n            break; // Segment found, safely exit the loop\n        }\n    }\n}"("vpp_val"=w1403, "voltages"="calibration values", "distances"="STROKE") -> ("stroke"=w1402:dbl)
    n1151 = local write "measured_stroke"(w1402) -> ()
    n1152 = local read "Quit"() -> (w1406:bool)
  }
  n1153 = while {
    shift-right: [w1420] -> w37
    shift-left: _ -> [w1411]
    shift-right: [w1419] -> w36
    shift-left: errorcluster {"status"=FALSE, "code"=0, "source"="Init"} ("error out") -> [w1413]
    tunnel: [w1408] -> w41
    tunnel: [w1418] -> _
    i -> [w1418]
    stop <- w1408 stop-if-true
    n1154 = local read "Com Port 2"() -> (w1412:refnum<visa-resource-name>)
    n1155 = local read "Port 2a"() -> (w1414:bool)
    n1156 = Unbundle(w1413) -> ("status"=→"Port 4":bool)  [unwired: 2 out]
    n1157 = call <vilib>:"High Resolution Polling Wait.vi"("seconds to wait"=0.02) -> ()  [unwired: 10 in, 1 out]
    n1158 = local read "Port 4"() -> (w1415:bool)
    n1159 = Not Equal?(x=w1412, y=w1411) -> (x != y?=w1410:bool)
    n1160 = Or(x=w1415, y=w1414) -> (x .or. y?=w1417:bool)
    n1161 = case shown="True" w1417 {
      frame False {
        w1423 = FALSE ("Visible")
        n1162 = property on="Port 2a" class="Bool (strict)"("Visible"=w1423) -> ()  [unwired: 2 in, 2 out]
        n1163 = property on="Port 4" class="Bool (strict)"("Visible"=w1423) -> ()  [unwired: 2 in, 2 out]
      }
      frame True {
        w1424 = TRUE ("Visible")
        n1164 = property on="Port 2a" class="Bool (strict)"("Visible"=w1424) -> ()  [unwired: 2 in, 2 out]
        n1165 = property on="Port 4" class="Bool (strict)"("Visible"=w1424) -> ()  [unwired: 2 in, 2 out]
      }
    }
    n1166 = case shown="True" w1410 {
      tunnel: [w1421 errorcluster {"status"=TRUE, "code"=0, "source"="Init"} ("error out")] -> w1409
      tunnel: w1413 -> [w1421 _]
      frame False {
      }
      frame True {
      }
    }
    n1167 = case shown="No Error" w1409 {
      selector: w1409 -> [w1435 w1466]
      tunnel: [w1428 w1471] -> w1420
      tunnel: [w1436 w1464] -> w1419
      tunnel: w1411 -> [w1438 w1469]
      frame No Error {
        n1168 = property class="Instr" props=["Serial Settings:Number of Bytes at Serial Port"](reference=w1438, error in=w1435) -> (reference out=w1429:refnum<visa-resource-name>, error out=w1434:errorcluster)  [unwired: 1 out]
        n1169 = while {
          tunnel: [w1446] -> w1430
          tunnel: [w1445] -> w1431
          tunnel: w1434 -> [w1444]
          tunnel: w1429 -> [w1443]
          tunnel: [w1442] -> _
          i -> [w1442]
          stop <- TRUE stop-if-true
          n1170 = property class="Instr" props=["Serial Settings:Number of Bytes at Serial Port"](reference=w1443, error in=w1444) -> (reference out=w1448:refnum<visa-resource-name>, error out=w1447:errorcluster)  [unwired: 1 out]
          n1171 = VISA Read(VISA resource name=w1448, byte count=u32 1000, error in (no error)=w1447) -> (VISA resource name out=w1445:refnum<visa-resource-name>, read buffer=→"Due read":string, error out=w1446:errorcluster)  [unwired: 1 out]
        }
        n1172 = local read "Command"() -> (w1426:string)
        n1173 = call <vilib>:"Trim Whitespace.vi"("string"=w1426) -> ("trimmed string"=w1425:string)  [unwired: 1 in]
        n1174 = Not Equal?(x=w1425, y="") -> (x != y?=w1432:bool)
        n1175 = case shown="True" w1432 {
          tunnel: w1431 -> [w1450 w1455]
          tunnel: [w1450 w1459] -> w1437
          tunnel: w1430 -> [w1449 w1454]
          tunnel: [w1449 w1457] -> w1436
          tunnel: w1425 -> [_ w1453]
          tunnel: [_ w1456] -> _
          frame False {
            # "DATA  WRITE LOOP"
          }
          frame True {
            n1176 = Concatenate Strings(w1453, "\r\n") -> (w1452:string)
            n1177 = VISA Write(VISA resource name=w1455, write buffer=w1452, error in (no error)=w1454) -> (VISA resource name out=w1459:refnum<visa-resource-name>, return count=w1456:u32, error out=w1458:errorcluster)
            n1178 = flat-sequence {
              tunnel: w1458 -> [w1461]
              tunnel: [w1461] -> w1457
              frame #0 {
                n1179 = local write "Command"("" ("Command")) -> ()
                n1180 = Wait (ms)(milliseconds to wait=u32 5) -> ()  [unwired: 1 out]
              }
            }
          }
        }
        n1181 = VISA Flush I/O Buffer(VISA resource name=w1437) -> (VISA resource name out=w1428:refnum<visa-resource-name>, error out=→"error out 9":errorcluster)  [unwired: 2 in]
      }
      frame Error {
        w1477 = u16 0 items=["None", "XON/XOFF", "RTS/CTS", "XON/XOFF & RTS/CTS", "DTR/DSR", "XON/XOFF & DTR/DSR"] ("flow control (0:none)  2")
        w1475 = u16 10 items=["1.0"=10, "1.5"=15, "2.0"=20] ("stop bits 2")
        w1473 = u16 0 items=["None", "Odd", "Even", "Mark", "Space"] ("parity 2")
        w1474 = u32 10000  # timeout (10sec)
        n1182 = VISA Clear(VISA resource name=w1469, error in (no error)=w1466) -> (VISA resource name out=w1468:refnum<visa-resource-name>, error out=w1467:errorcluster)
        n1183 = VISA Close(VISA resource name=w1468, error in (no error)=w1467) -> (error out=w1470:errorcluster)
        n1184 = call <vilib>:"Clear Errors.vi"("error in (no error)"=w1470) -> ()  [unwired: 5 in, 2 out]
        n1185 = local read "Com Port 2"() -> (w1463:refnum<visa-resource-name>)
        "visa due" <- w1463
        n1186 = call-poly "VISA Configure Serial Port"("VISA resource name"=w1463, "timeout (10sec)"=w1474, "baud rate (9600)"=u32 250000 ("baud rate  2"), "data bits (8)"=u16 8 ("data bits  2"), "parity (0:none)"=w1473, "stop bits (10: 1 bit)"=w1475, "flow control (0:none)"=w1477) -> ("VISA resource name out"=w1478:refnum<visa-resource-name>, "error out"=w1479:errorcluster)  [unwired: 7 in]
        n1187 = flat-sequence {
          tunnel: w1478 -> [w1481]
          tunnel: w1479 -> [w1480]
          tunnel: [w1481] -> w1471
          tunnel: [w1480] -> w1464
          frame #0 {
            n1188 = Wait (ms)(milliseconds to wait=u32 50) -> ()  [unwired: 1 out]
          }
        }
        "Residual Due" <- ""
        "Port 2 Error" <- w1464
      }
    }
    n1189 = local read "Quit"() -> (w1408:bool)
    "Error Due" <- w1413
  }
  n1190 = local write "FRICVALZ"(0.0 ("FRICVALZ")) -> ()
  n1191 = property on="RUN" class="Bool (strict)"("Visible"=TRUE) -> ()  [unwired: 2 in, 2 out]
  n1192 = while {
    tunnel: [w1498] -> _
    tunnel: [w1483] -> w54
    i -> [w1498]
    stop <- w1483 stop-if-true
    n1193 = local read "conststatus"() -> (w1487:dbl)
    n1194 = local read "Main Tab"() -> (w1485:T2)
    n1195 = local read "EDIT"() -> (w1504:bool)
    n1196 = local read "Rate"() -> (w1503:dbl)
    n1197 = case shown="True" w1504 {
      tunnel: [FALSE TRUE] -> w1490
      frame False {
      }
      frame True {
      }
    }
    n1198 = property on="Time slide" class="Slide (strict)"("Scale.Range:Maximum"=2500.0) -> ()  [unwired: 2 in, 2 out]
    n1199 = Equal?(x=w1485, y=T20."About" ("Main Tab")) -> (x = y?=w1496:bool)
    n1200 = Equal?(x=w1487, y=0.0) -> (x = y?=w1488:bool)
    n1201 = Divide(x=1.0, y=w1503) -> (x/y=w1499:dbl)
    "Time 2" <- w1499
    n1202 = case shown="True" w1488 {
      frame False {
      }
      frame True {
        # "C:\\WinDucom\\calibrate WO 2391.dcf"
        n1203 = local write "Lan flag"(22) -> ()
        n1204 = local write "conststatus"(10.0 ("rpm value : 2")) -> ()
        n1205 = String To Path(string="C:\\LAB-IQ\\calibrate WO 2465.dcf") -> (path=w1510:path)
        n1206 = Open/Create/Replace File "Open File"(file path (use dialog)=w1510) -> (refnum out=w1508:refnum<file>)  [unwired: 5 in, 2 out]
        n1207 = for {
          N: 23 -> [_]
          tunnel: w1508 -> [w1519]
          i -> [w1513]
          (unwired) TRUE ("line mode (F)")
          n1208 = Read from Text File "Read File"(file (use dialog)=w1519) -> (text=w1518:string)  [unwired: 3 in, 3 out]
          n1209 = Match Pattern(string=w1518, regular expression="]") -> (after substring=w1516:string)  [unwired: 1 in, 3 out]
          n1210 = String Subset(string=w1518, offset (0)=5, length (rest)=10 ("length (rest)")) -> (substring=w1511:string)
          n1211 = Fract/Exp String To Number(string=w1511) -> (number=w1512:dbl)  [unwired: 3 in, 1 out]
          n1212 = Match Pattern(string=w1516, regular expression="-") -> (before substring=w1514:string)  [unwired: 1 in, 3 out]
          n1213 = case shown="5" w1513 {
            tunnel: w1512 -> [w1522 w1523 w1524 w1525 _ _ _ w1530 w1531 _ w1532 w1533 w1534 w1535 w1536 w1537 _ w1538 w1539 _ _ _ _ _]
            tunnel: w1514 -> [_ _ _ _ w1526 w1527 w1528 _ _ _ _ _ _ _ _ _ _ _ _ w1540 w1541 _ w1542 _]
            frame 0 {
              n1214 = local write "FRIC. FORCE :"(w1522) -> ()
            }
            frame 1 {
              n1215 = local write "TEMPERATURE :"(w1523) -> ()
            }
            frame 2 {
              n1216 = local write "HUMIDITY:"(w1524) -> ()
            }
            frame 3 {
              n1217 = local write "AIR TEMPERATURE :"(w1525) -> ()
            }
            frame 4 {
              n1218 = local write "Com Port 1"(w1526) -> ()
            }
            frame 5 {
              n1219 = local write "Com Port 2"(w1527) -> ()
              n1220 = local write "visa due"(w1527) -> ()
            }
            frame 6 {
              n1221 = String To Path(string=w1528) -> (path=w1529:path)
              n1222 = local write "File Path"(w1529) -> ()
              "String" <- w1528
            }
            frame 7 {
              n1223 = local write "DISPLACEMENT :"(w1530) -> ()
            }
            frame 8 {
              n1224 = local write "STROKE GAIN :"(w1531) -> ()
            }
            frame 9 {
            }
            frame 10 {
              n1225 = local write "Language Selection"(w1532) -> ()
            }
            frame 11 {
              n1226 = local write "CH-POWER +"(w1533) -> ()
            }
            frame 12 {
              n1227 = local write "CH-POWER -"(w1534) -> ()
            }
            frame 13 {
              n1228 = local write "CH-HEATER"(w1535) -> ()
            }
            frame 14 {
              n1229 = local write "CH-HUMIDITY WET"(w1536) -> ()
            }
            frame 15 {
              n1230 = local write "CH-HUMIDITY DRY"(w1537) -> ()
            }
            frame 16 {
            }
            frame 17 {
              n1231 = local write "AIR TEMP INTERCEPT:"(w1538) -> ()
            }
            frame 18 {
              n1232 = local write "TEMP INTERCEPT:"(w1539) -> ()
            }
            frame 19 {
              n1233 = local write "S.NO"(w1540) -> ()
            }
            frame 20 {
              n1234 = local write "Com Port 3"(w1541) -> ()
            }
            frame 21 {
            }
            frame 22 {
              n1235 = local write "C3 :"(w1542) -> ()
            }
            frame 23, Default {
            }
          }
        }
      }
    }
    n1236 = Select(t=u32 2500 ("milliseconds to wait"), s=w1496, f=u32 500 ("milliseconds to wait")) -> (s? t:f=w1494:u32)
    n1237 = Multiply(x=w1499, y=w1494) -> (x*y=w1501:dbl)
    n1238 = property on="Time slide" class="Slide (strict)"("Visible"=w1490) -> ()  [unwired: 2 in, 2 out]
    n1239 = call "Elapsed Time2"("Time Target (s)"=w1501, "Auto Reset"=TRUE) -> ("Time has Elapsed"=w1491:bool)  [unwired: 10 in, 7 out]
    n1240 = case shown="True" w1491 {
      frame False {
      }
      frame True {
        n1241 = stacked-sequence {
          frame #0 {
            w1543 = 0.0
            # "DATA PROCESSING"
            # "115 mV/N"
            n1242 = local read "RH Numeric:"() -> (w1549:dbl)
            n1243 = local read "HUMIDITY:"() -> (w1550:dbl)
            n1244 = local read "FRICVALZ"() -> (w1561:dbl)
            n1245 = local read "Friction"() -> (w1544:dbl)
            n1246 = local write "TEMP"(w1543) -> ()
            n1247 = Multiply(x=w1549, y=w1550) -> (x*y=→"Humidity ( %RH )" →"Hum" →"Hum 2":dbl)
            n1248 = Subtract(x=w1544, y=w1561) -> (x-y=w1556:dbl)
            "FF 2" <- w1556
            "FF 4" <- w1556
            n1249 = local read "TEMP"() -> (w1560:dbl)
            n1250 = local write "FF 3"(w1556) -> ()
            n1251 = Compound Arithmetic op=OR("FRICVALZ 4", "FRICVALZ 3", "FRICVALZ 2") -> (w1552:bool)
            n1252 = case shown="True" w1552 {
              tunnel: w1544 -> [_ w1567]
              frame False {
              }
              frame True {
                w1566 = FALSE ("FRICVALZ")
                n1253 = local write "FRICVALZ 3"(w1566) -> ()
                n1254 = local write "FRICVALZ 2"(w1566) -> ()
                n1255 = local write "FRICVALZ 4"(w1566) -> ()
                "FRICVALZ" <- w1567
              }
            }
            n1256 = Not A Number/Path/Refnum?(number/path/refnum=w1560) -> (NaN/Path/Refnum?=w1559:bool)
            n1257 = Not A Number/Path/Refnum?(number/path/refnum=w1556) -> (NaN/Path/Refnum?=w1558:bool)
            n1258 = Divide(x=w1556, y=1.96) -> (x/y=w1553:dbl)
            n1259 = Compound Arithmetic op=OR(w1559, w1558) -> (w1557:bool)
            n1260 = Not A Number/Path/Refnum?(number/path/refnum=w1553) -> (NaN/Path/Refnum?=w1554:bool)
            n1261 = case shown="True" w1557 {
              frame False {
              }
              frame True {
                n1262 = local write "TEMP"(0.0 ("TEMP")) -> ()
                n1263 = local write "FF 2"(0.0 ("FF 2")) -> ()
                n1264 = local write "reinit"(TRUE ("reinit")) -> ()
              }
            }
            n1265 = Select(t=0.0, s=w1554, f=w1553) -> (s? t:f=→"COF 2":dbl)
            "AIR TEMP" <- w1543
            "TEMP 2" <- w1543
            "TEMP 3" <- w1543
          }
        }
      }
    }
    n1266 = Wait (ms)(milliseconds to wait=u32 50) -> ()  [unwired: 1 out]
    n1267 = local read "Quit"() -> (w1483:bool)
    "Rate" <- 2500.0 ("No of Samples")
  }
  n1268 = while {
    tunnel: w57 -> [_]
    tunnel: [w1594] -> _
    tunnel: [w1570] -> w56
    i -> [w1594]
    stop <- w1570 stop-if-true
    # "C:\\LAB-IQ-NXT\\Scar View.exe"
    n1269 = local read "OK Button 16"() -> (w1583:bool)
    n1270 = local read "Main Tab"() -> (w1576:T2)
    n1271 = local read "service 3"() -> (w1577:bool)
    n1272 = local read "OPEN 6"() -> (w1579:bool)
    n1273 = local read "EDIT 2"() -> (w1581:bool)
    n1274 = flat-sequence {
      frame #0 {
        n1275 = local read "SAVE 2"() -> (w2196:bool)
        n1276 = stacked-sequence {
          frame #0 {
            n1277 = local read "EDIT"() -> (w2250:bool)
            n1278 = case shown="True" w2250 {
              tunnel: [u8 2 ("Disabled") u8 0 ("Disabled")] -> _
              frame False {
                w2252 = FALSE
                n1279 = local write "Password"("") -> ()
                n1280 = property on="SrvM CP" class="Bool (strict)"("Visible"=w2252) -> ()  [unwired: 2 in, 2 out]
                n1281 = property on="message" class="Str"("Visible"=w2252) -> ()  [unwired: 2 in, 2 out]
                n1282 = local write "x = y?"(w2252) -> ()
                n1283 = property on="Password" class="Str"("Visible"=w2252) -> ()  [unwired: 2 in, 2 out]
                n1284 = property on="ENTER THE NEW PASSWORD" class="Str"("Visible"=w2252) -> ()  [unwired: 2 in, 2 out]
                n1285 = property on="ENTER CURRENT PASSWORD" class="Str"("Visible"=w2252) -> ()  [unwired: 2 in, 2 out]
                n1286 = local write "SrvM CP"(w2252) -> ()
              }
              frame True {
                w2255 = TRUE
                n1287 = property on="SrvM CP" class="Bool (strict)"("Visible"=w2255) -> ()  [unwired: 2 in, 2 out]
                n1288 = property on="Password" class="Str"("Visible"=w2255) -> ()  [unwired: 2 in, 2 out]
              }
            }
            "dipl pwd" <- "@143$\n" ("dipl pwd")
          }
          frame #1 {
            # "Gain password"
            n1289 = String To Byte Array(string="ENTER CURRENT PASSWORD") -> (unsigned byte array=w2260:u8[])
            n1290 = Search 1D Array(1D array=w2260, element=u8 10) -> (index of element=w2263:i32)  [unwired: 1 in]
            n1291 = Index Array(array=w2260, index=w2263) -> (element=w2259:u8)
            n1292 = Equal?(x=w2259, y=10) -> (x = y?=w2257:bool)
            n1293 = case shown="True" w2257 {
              frame False {
